vi "SetSourceOutputEnableAction.vi"(7 "SMU":T1, 8 "Error In":errorcluster, 10 "Enable?":bool, 11 "Keithley 2602 In":refnum<visa-resource-name>) -> (0 "Error Out":errorcluster, 3 "Keithley 2602 Out":refnum<visa-resource-name>)   [LabVIEW 2012, in "Keithley-2602.lvlib"]
uses:
  Keithley-2602.lvlib
  Controls/SMU.ctl
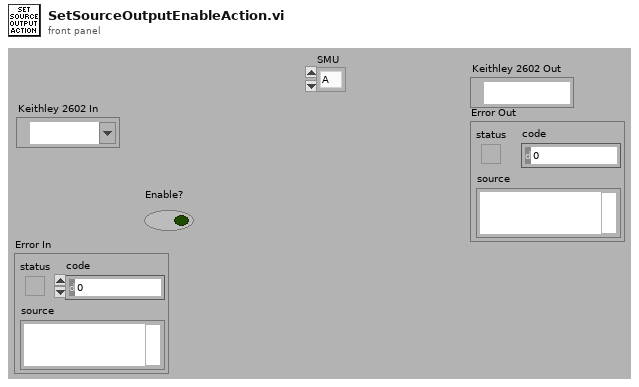
[diagram p1: front panel]
types:
  T1 = typedef "Keithley-2602.lvlib/SMU.ctl" = enum16{"A", "B"}
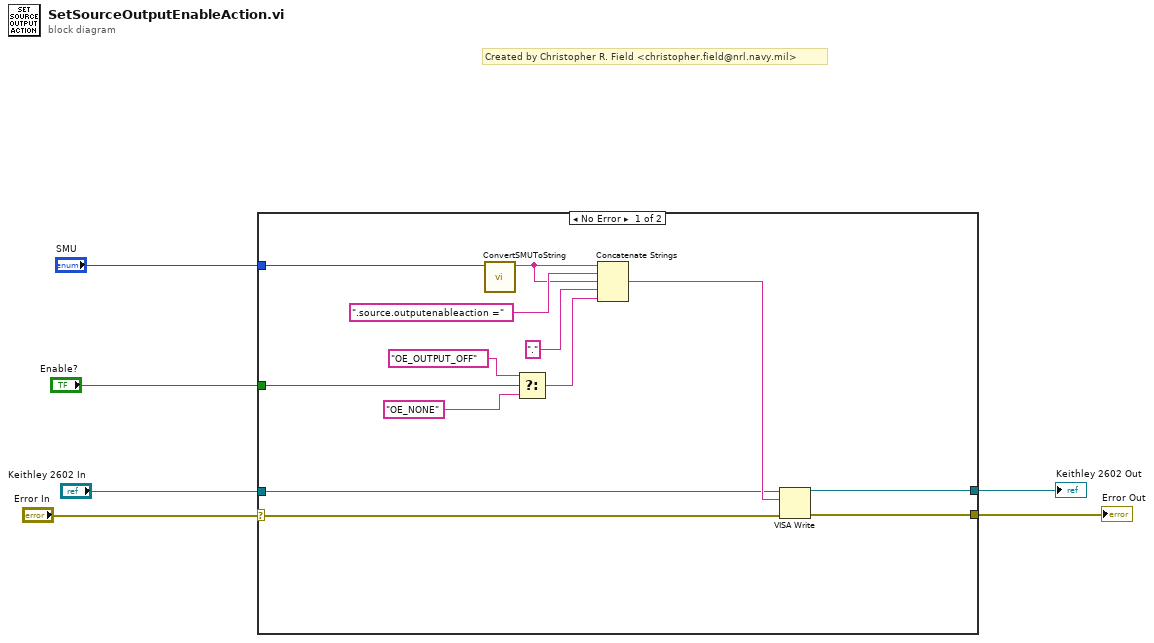
[diagram p0: block diagram]
diagram:
  # "Created by Christopher R. Field <christopher.field@nrl.navy.mil>"
  n1 = case shown="No Error" "Error In" {
    selector: "Error In" -> [w7 w20]
    tunnel: "Enable?" -> [w19 _]
    tunnel: "Keithley 2602 In" -> [w14 w21]
    tunnel: [w13 w21] -> w4
    tunnel: [w12 w20] -> w3
    tunnel: "SMU" -> [w8 _]
    frame No Error {
      n2 = call "ConvertSMUToString.vi"("SMU"=w8) -> ("Channel"=w11:string)  [unwired: 10 in]
      n3 = Select(t="OE_OUTPUT_OFF", s=w19, f="OE_NONE") -> (s? t:f=w9:string)
      n4 = Concatenate Strings(w11, ".source.outputenableaction =", w11, "." ("string"), w9) -> (w15:string)
      n5 = VISA Write(VISA resource name=w14, write buffer=w15, error in (no error)=w7) -> (VISA resource name out=w13:refnum<visa-resource-name>, error out=w12:errorcluster)  [unwired: 1 out]
    }
    frame Error {
    }
  }
  "Keithley 2602 Out" <- w4
  "Error Out" <- w3
